vi "Traitement 1 cible.vi"(9 "Indications Pokaenmon D":T2, 11 "Indications Pokaenmon G":T2) -> (0 "D détect":bool, 1 "G détect":bool, 2 "Données caméras":T1, 3 "Distance":string, 4 "Signature":u32)   [LabVIEW 2013]
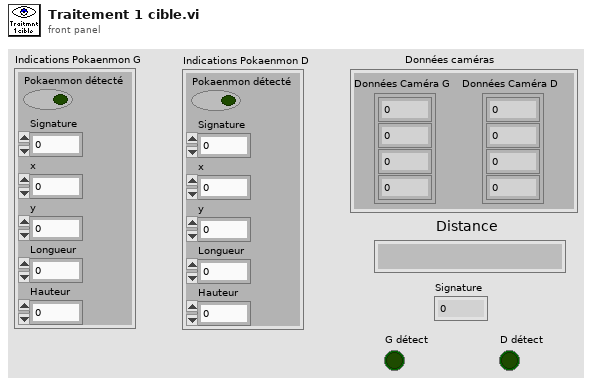
[diagram p1: front panel]
types:
  T1 = cluster{"Données Caméra G":cluster{dbl, dbl, dbl, dbl}, "Données Caméra D":cluster{dbl, dbl, dbl, dbl}}
  T2 = cluster{"Pokaenmon détecté":bool, "Signature":u32, "x":dbl, "y ":dbl, "Longueur":dbl, "Hauteur":dbl}
  T3 = cluster{cluster{dbl, dbl, dbl, dbl}, cluster{dbl, dbl, dbl, dbl}}
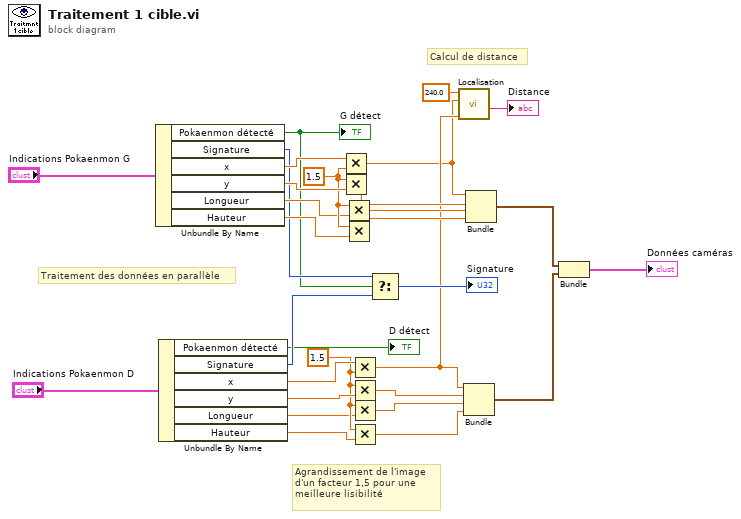
[diagram p0: block diagram]
diagram:
  w19 = 1.5
  w24 = 1.5
  # "Agrandissement de l'image\nd'un facteur 1,5 pour une \nmeilleure lisibilité"
  # "Traitement des données en parallèle"
  # "Calcul de distance"
  n1 = Unbundle By Name("Indications Pokaenmon G") -> ("Pokaenmon détecté"=w4:bool, "Signature"=w13:u32, "x"=w28:dbl, "y"=w29:dbl, "Longueur"=w22:dbl, "Hauteur"=w23:dbl)
  "G détect" <- w4
  n2 = Unbundle By Name("Indications Pokaenmon D") -> ("Pokaenmon détecté"=→"D détect":bool, "Signature"=w12:u32, "x"=w20:dbl, "y"=w21:dbl, "Longueur"=w17:dbl, "Hauteur"=w18:dbl)
  n3 = Multiply(x=w28, y=w24) -> (x*y=w9:dbl)
  n4 = Multiply(x=w24, y=w29) -> (x*y=w27:dbl)
  n5 = Multiply(x=w24, y=w22) -> (x*y=w25:dbl)
  n6 = Multiply(x=w24, y=w23) -> (x*y=w26:dbl)
  n7 = Multiply(x=w20, y=w19) -> (x*y=w10:dbl)
  n8 = Multiply(x=w19, y=w21) -> (x*y=w16:dbl)
  n9 = Multiply(x=w19, y=w17) -> (x*y=w15:dbl)
  n10 = Multiply(x=w19, y=w18) -> (x*y=w14:dbl)
  n11 = Select(t=w13, s=w4, f=w12) -> (s? t:f=→"Signature":u32)
  n12 = call "Localisation.vi"("x2"=w10, "x1"=w9, "b"=240.0) -> ("d"=→"Distance":string)  [unwired: 8 in]
  n13 = Bundle(w10, w16, w15, w14) -> (w2:cluster{dbl, dbl, dbl, dbl})  [unwired: 1 in]
  n14 = Bundle(w9, w27, w25, w26) -> (w3:cluster{dbl, dbl, dbl, dbl})  [unwired: 1 in]
  n15 = Bundle(w3, w2) -> (→"Données caméras":T3)  [unwired: 1 in]
